vi "Get VISA gRPC Open Close Behavior.vi"(0 "initialize session behavior":T2, 11 "error in (no error)":errorcluster) -> (4 "open/close behavior":T1, 15 "error out":errorcluster)   [LabVIEW 2021, in "KeysightDmm.lvclass"]
uses:
  KeysightDmm.lvclass
  <vilib>/Plug-In SDKs/Sessions/Instrument/ISession Factory/Initialize and Close Session Behavior.ctl
  <vilib>/NI-VISA/VISA gRPC Open Close Behavior.ctl
  <vilib>/Plug-In SDKs/Sessions/Instrument/ISession Factory/ISession Factory.lvclass
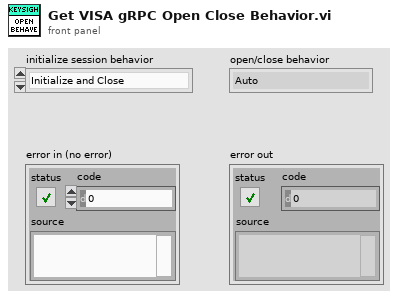
[diagram p1: front panel]
types:
  T1 = typedef "VISA gRPC Open Close Behavior.ctl" = enum16{"Auto", "Initialize and Close", "Attach and Detach", "Initialize and Detach", "Attach and Close"}
  T2 = typedef "NI Session Management Instrument.lvlib/ISession Factory.lvclass/Initialize and Close Session Behavior.ctl" = enum16{"Initialize and Close", "Attach and Detach", "Initialize and Detach", "Attach and Close"}
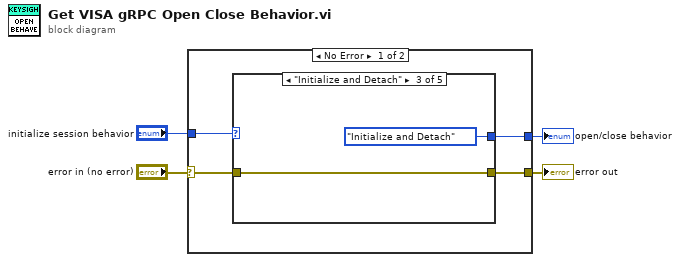
[diagram p0: block diagram]
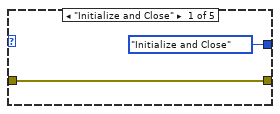
[diagram p2: hidden frame]
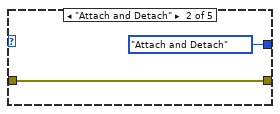
[diagram p3: hidden frame]
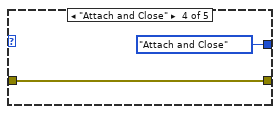
[diagram p4: hidden frame]
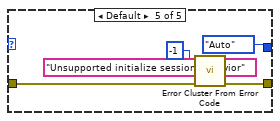
[diagram p5: hidden frame]
diagram:
  n1 = case shown="No Error" "error in (no error)" {
    selector: "error in (no error)" -> [w5 w22]
    tunnel: "initialize session behavior" -> [w8 _]
    tunnel: [w7 _] -> w3
    tunnel: [w6 w22] -> w2
    frame No Error {
      n2 = case shown="\"Initialize and Detach\"" w8 {
        tunnel: [VISA_gRPC_Open_Close_Behavior."Initialize and Close" ("open/close behavior") VISA_gRPC_Open_Close_Behavior."Attach and Detach" ("open/close behavior") VISA_gRPC_Open_Close_Behavior."Initialize and Detach" ("open/close behavior") VISA_gRPC_Open_Close_Behavior."Attach and Close" ("open/close behavior") VISA_gRPC_Open_Close_Behavior."Auto" ("open/close behavior")] -> w7
        tunnel: [w9 w11 w13 w15 w20] -> w6
        tunnel: w5 -> [w9 w11 w13 w15 w21]
        frame "Initialize and Close" {
        }
        frame "Attach and Detach" {
        }
        frame "Initialize and Detach" {
        }
        frame "Attach and Close" {
        }
        frame Default {
          n3 = call <vilib>:"Error Cluster From Error Code.vi"("error in (no error)"=w21, "error message (\"\")"="Unsupported initialize session behavior" ("error message (\"\")"), "error code (0)"=-1) -> ("error out"=w20:errorcluster)  [unwired: 6 in]
        }
      }
    }
    frame Error {
    }
  }
  "open/close behavior" <- w3
  "error out" <- w2
